vi "AlazarSetLED.vi"(3 "error in (no error)":errorcluster, 4 "State":bool, 5 "Handle":u64) -> (0 "error out":errorcluster, 1 "Return Code":u32, 2 "Handle":u64)   [LabVIEW 2018]
doc: "Control LED on a board's PCI/PCIe mounting bracket."
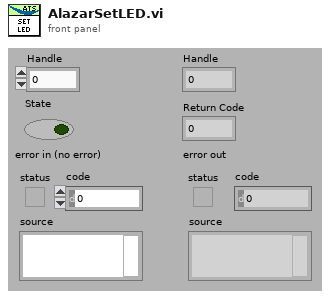
[diagram p1: front panel]
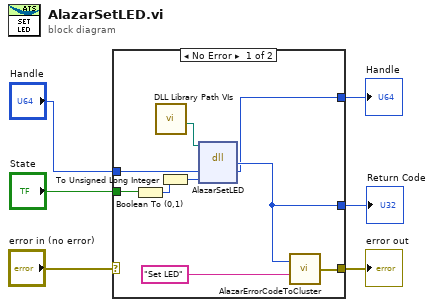
[diagram p0: block diagram]
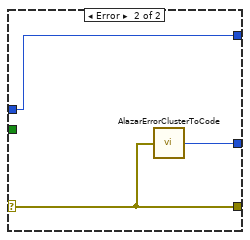
[diagram p2: hidden frame]
diagram:
  n1 = case shown="No Error" "error in (no error)" {
    selector: "error in (no error)" -> [_ w18]
    tunnel: [w12 w18] -> w5
    tunnel: [w14 w17] -> w4
    tunnel: "Handle" -> [w15 w16]
    tunnel: [w11 w16] -> w2
    tunnel: "State" -> [w10 _]
    frame No Error {
      n2 = Boolean To (0,1)(Boolean=w10) -> (0, 1=w9:i16)
      n3 = call "DLL Library Path VIs.vi"() -> ("Alazar"=w7:path)  [unwired: 9 in, 2 out]
      n4 = To Unsigned Long Integer(number=w9) -> (unsigned 32bit integer=w8:u32)
      n5 = dll-call lib="C:/Project/SerialSectOCT - FFT GPU/SerialSectOCT/Labview Software/DLL/ATSApi.dll" fn="AlazarSetLED"(path in=w7, "handle"=w15, "ledON"=w8) -> ("return type"=w14:u32, "handle"=w11:u64)  [unwired: 3 in, 2 out]
      n6 = call "AlazarErrorCodeToCluster.vi"("Message"="Set LED", "Error Code"=w14) -> ("error out"=w12:errorcluster)
    }
    frame Error {
      n7 = call "AlazarErrorClusterToCode.vi"("error in (no error)"=w18) -> ("Error Code"=w17:u32)
    }
  }
  "Handle" <- w2
  "error out" <- w5
  "Return Code" <- w4
